vi "UiGasMeasurement.vi"() -> ()   [LabVIEW 2011]
uses:
  Output - Cluster b2g1.ctl
  <vilib>/Platform/TimedLoop/XDataNode/timing_clust.ctl
  <vilib>/Platform/TimedLoop/XDataNode/nitl_modes.ctl
  <vilib>/Platform/TimedLoop/XDataNode/wakeup.ctl
  <vilib>/Instr/_visa.llb/VISA Configure Serial Port (Instr).vi
  <vilib>/Platform/TimedLoop/XDataNode/XDataNode.xnode
  <vilib>/Platform/TimedLoop/XDataNode/XDNodeRunTimeDep.lvlib
panel:
  out "Verlauf":T1(graph)
  out "pump":bool
  out "timestamp 2":timestamp
  out "log":string[](array[string])
  out "h2":dbl
  out "ch4":dbl
  out "co2":dbl
  out "timestamp":timestamp
  out "return count":u32
  out "read string":string
  out "Volumen [l]":dbl format="%.2f"
  in  "stop":bool
  out "TS-6 [°C]":dbl format="%.2g"
  out "DS-3 [bar]":dbl format="%.5g"
  # "#MS 26.07.12 15:36:48    21.98 Vol% CO2  72.54 Vol% CH4   1.05 Vol% H2\n\n#AL 27.07.12 16:34:22  37 EIN externe Pumpe \n\n#AL 27.07.12 16:40:29  37 AUS externe Pumpe"
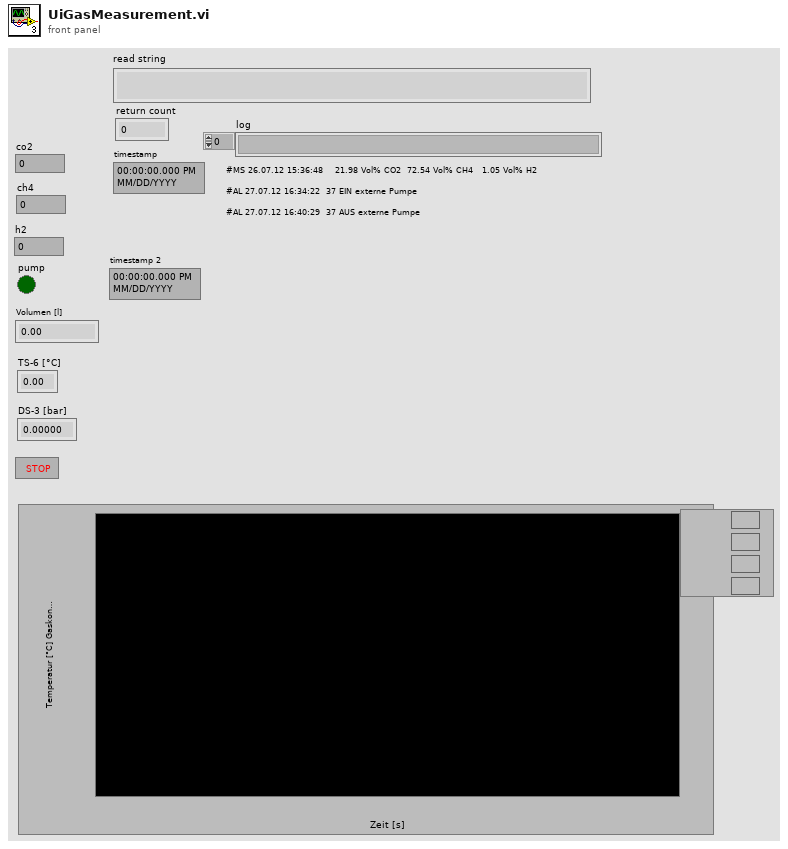
[diagram p1: front panel]
types:
  T1 = cluster{"co2 [%]":dbl, "ch4 [%]":dbl, "h2 [%]":dbl, "TS-6 [°C]":dbl}
  T2 = cluster{"ch4 [%]":dbl, "co2 [%]":dbl, "h2 [%]":dbl, "pump":bool, "log":string[], "Volumen [l]":dbl, "TS-6 [°C]":dbl, "DS-3 [bar]":dbl}
  T3 = typedef "Output - Cluster b2g1.ctl" = cluster{"DFS-1 [dl]":u64, "FS-3 [l]":dbl, "DFS-1 [l/min]":dbl, "DS-1 [bar]":dbl, "V-10 ZU":bool, "V-14 ZU":bool, "FS-1 [l]":dbl, "FS-2 [l]":dbl, "TS-4 [°C]":dbl, "HS-1":bool, "V-13 [%]":u8, "V-15 [%]":u8, "P-4 [%]":u8, "P-5 [%]":u8, "Dosierung":bool, "MR Max Füllstand":bool, "MR Min Füllstand":bool, "Dosiermenge [l]":sgl, "V-14 AUF":bool, "V-10 AUF":bool, "T-1 Max Füllstand":bool, "T-1 Min Füllstand":bool, "T-2 Max Füllstand":bool, "T-2 Min Füllstand":bool, "pHS-1 [pH]":dbl, "P-4 RUN":bool, "P-5 RUN ":bool, "V-33 AUF":bool, "V-33 ZU":bool, "V-34 AUF":bool, "V-34 ZU":bool, "P-4 ERR":bool, "P-5 ERR":bool, "TS-5 [°C]":dbl, "GZ-1 [dl]":u64, "TS-6 [°C]":dbl, "DS-3 [bar]":dbl}
  T4 = typedef "XDNodeRunTimeDep.lvlib/timing_clust.ctl" = cluster{"Expected End [f-1]":u64, "Actual End [f-1]":u64, "Finished Late? [f-1]":bool, "Expected End [i-1]":u64, "Actual End [i-1]":u64, "Finished Late? [i-1]":bool, "Expected Start [i]":u64, "Actual Start [i]":u64, "Expected Start [f]":u64, "Actual Start [f]":u64, "Source Name":string, "Structure Name":string, "Period":i64, "Deadline":i64, "Offset":i64, "Start":i64, "Priority":i32, "Timeout":i32, "Mode":T5, "Wakeup Reason":T6, "Error":errorcluster, "Source Type":string, "Secondary Source Type":string, "Global End Time":u64, "Global Start Time":u64, "Frame Duration":u64, "Iteration Duration":u64, "Assigned CPU":i32, "I/O Scan Engine Mode":u32}
  T5 = typedef "XDNodeRunTimeDep.lvlib/nitl_modes.ctl" = enum32{"No Change", "Process missed periods, maintain original phase", "Discard missed periods, maintain original phase", "Process missed periods, ignore original phase", "Discard missed periods, ignore original phase"}
  T6 = typedef "XDNodeRunTimeDep.lvlib/wakeup.ctl" = enum32{"Normal", "Aborted", "Asynchronous wakeup", "Timing source error", "Timed loop error", "Timeout"}
  T7 = enum32{"invalid app kind", "Development System", "Run Time System", "Student Edition", "Embedded LabVIEW", "Evaluation", "Custom"}
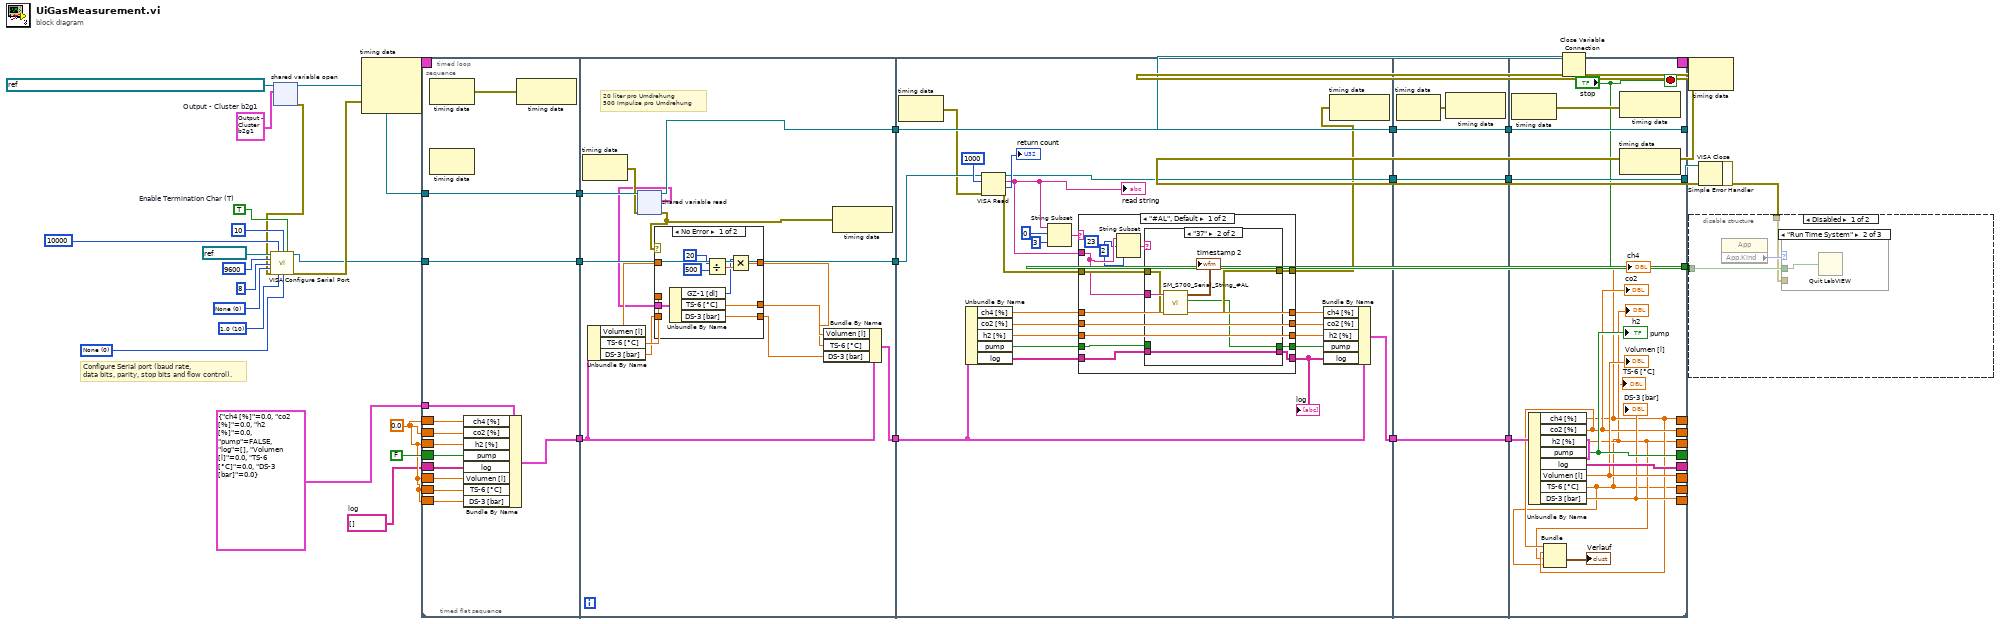
[diagram p0: block diagram]
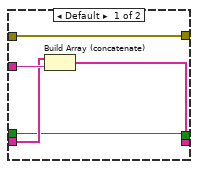
[diagram p6: hidden frame]
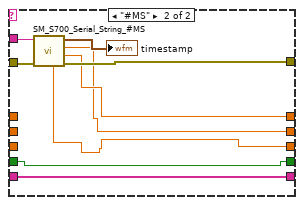
[diagram p7: hidden frame]
diagram:
  w1 = string[] []  # log
  w2 = 0.0 ("co2")
  w17 = u16 0 items=["None", "Odd", "Even", "Mark", "Space"] ("parity")
  w14 = u16 10 items=["1.0"=10, "1.5"=15, "2.0"=20] ("stop bits")
  w13 = u16 0 items=["None"=0, "XON/XOFF"=1, "RTS/CTS"=2, "DTR/DSR"=4] ("flow control")
  w15 = TRUE  # Enable Termination Char (T)
  w26 = T3 {"DFS-1 [dl]"=0, "FS-3 [l]"=0.0, "DFS-1 [l/min]"=0.0, "DS-1 [bar]"=0.0, "V-10 ZU"=FALSE, "V-14 ZU"=FALSE, "FS-1 [l]"=0.0, "FS-2 [l]"=0.0, "TS-4 [°C]"=0.0, "HS-1"=FALSE, "V-13 [%]"=0, "V-15 [%]"=0, "P-4 [%]"=0, "P-5 [%]"=0, "Dosierung"=FALSE, "MR Max Füllstand"=FALSE, "MR Min Füllstand"=FALSE, "Dosiermenge [l]"=0.0, "V-14 AUF"=FALSE, "V-10 AUF"=FALSE, "T-1 Max Füllstand"=FALSE, "T-1 Min Füllstand"=FALSE, "T-2 Max Füllstand"=FALSE, "T-2 Min Füllstand"=FALSE, "pHS-1 [pH]"=0.0, "P-4 RUN"=FALSE, "P-5 RUN "=FALSE, "V-33 AUF"=FALSE, "V-33 ZU"=FALSE, "V-34 AUF"=FALSE, "V-34 ZU"=FALSE, "P-4 ERR"=FALSE, "P-5 ERR"=FALSE, "TS-5 [°C]"=0.0, "GZ-1 [dl]"=0, "TS-6 [°C]"=0.0, "DS-3 [bar]"=0.0}  # Output - Cluster b2g1
  # "Configure Serial port (baud rate,\ndata bits, parity, stop bits and flow control)."
  n1 = shared-variable-open(refnum<k21> "ni.var.psp://10.27.40.24/variables - b2g1/data - network - b2g1" ("shared variable refnum in"), w26) -> (w27:refnum<k21>, w10:errorcluster)  [unwired: 2 in]
  n2 = call-poly "VISA Configure Serial Port"("VISA resource name"=refnum<visa-resource-name> "COM1", "timeout (10sec)"=u32 10000, "termination char\n(0xA = '\\n' = LF)"=u8 10 ("termination char\n(0xA = '\\n' = LF)"), "Enable Termination\nChar (T)"=w15, "baud rate (9600)"=u32 9600 ("baud rate"), "data bits (8)"=u16 8 ("data bits"), "parity (0:none)"=w17, "error in (no error)"=w10, "stop bits (10: 1 bit)"=w14, "flow control (0:none)"=w13) -> ("VISA resource name out"=w6:refnum<visa-resource-name>, "error out"=w9:errorcluster)  [unwired: 4 in]
  n3 = node-c288(w9) -> (w25:T4)  [unwired: 2 in]
  n4 = timed-loop {
    timing: w25 -> [_]
    timing-out: [_] -> w24
    tunnel: w27 -> [w50]
    tunnel: [w49] -> w22
    tunnel: [w48] -> w21
    tunnel: w6 -> [w47]
    tunnel: [w46] -> w5
    shift-right: [w45] -> _
    shift-left: w1 -> [w44]
    tunnel: T2 {"ch4 [%]"=0.0, "co2 [%]"=0.0, "h2 [%]"=0.0, "pump"=FALSE, "log"=[], "Volumen [l]"=0.0, "TS-6 [°C]"=0.0, "DS-3 [bar]"=0.0} ("Cluster") -> [w43]
    shift-right: [w42] -> _
    shift-left: w2 -> [w41]
    shift-right: [w40] -> _
    shift-left: w2 -> [w39]
    shift-right: [w38] -> _
    shift-left: w2 -> [w37]
    shift-right: [w36] -> _
    shift-left: FALSE ("pump") -> [w35]
    shift-right: [w34] -> _
    shift-left: w2 -> [w33]
    shift-right: [w32] -> _
    shift-left: w2 -> [w31]
    shift-right: [w30] -> _
    shift-left: w2 -> [w29]
    stop <- "stop" stop-if-true
    n5 = timed-sequence {
      timing: _ -> [_]
      timing-out: _ -> [_]
      tunnel: w50 -> [w84]
      tunnel: [w83] -> w49
      tunnel: [w82] -> w48
      tunnel: w47 -> [w79]
      tunnel: [w78] -> w46
      tunnel: [w77] -> w45
      tunnel: w44 -> [w76]
      tunnel: w43 -> [w73]
      tunnel: [w70] -> w42
      tunnel: w41 -> [w69]
      tunnel: [w68] -> w40
      tunnel: w39 -> [w67]
      tunnel: [w66] -> w38
      tunnel: w37 -> [w65]
      tunnel: [w64] -> w36
      tunnel: w35 -> [w63]
      tunnel: [w62] -> w34
      tunnel: w33 -> [w61]
      tunnel: [w60] -> w32
      tunnel: w31 -> [w59]
      tunnel: [w58] -> w30
      tunnel: w29 -> [w57]
      n6 = timed-flat-sequence {
        tunnel: w76 -> [w88]
        tunnel: w79 -> [w96]
        tunnel: w84 -> [w97]
        tunnel: [w97] -> w75
        tunnel: [w96] -> w74
        tunnel: w73 -> [w94]
        tunnel: [w93] -> w71
        tunnel: w69 -> [w92]
        tunnel: w67 -> [w91]
        tunnel: w65 -> [w90]
        tunnel: w63 -> [w89]
        tunnel: w61 -> [w85]
        tunnel: w59 -> [w86]
        tunnel: w57 -> [w87]
        tunnel: [w114] -> w81
        tunnel: [w113] -> w80
        tunnel: w75 -> [w116]
        tunnel: w74 -> [w113]
        tunnel: [w111] -> w72
        tunnel: w71 -> [w110]
        tunnel: w81 -> [w156]
        tunnel: w80 -> [w153]
        tunnel: w72 -> [w143]
        tunnel: [w156] -> w56
        tunnel: [w152] -> w54
        tunnel: [w142] -> w52
        tunnel: w56 -> [w198]
        tunnel: [w198] -> w55
        tunnel: w54 -> [w197]
        tunnel: [w197] -> w53
        tunnel: w52 -> [w196]
        tunnel: [w196] -> w51
        tunnel: [w211] -> w64
        tunnel: [w205] -> w66
        tunnel: [w207] -> w68
        tunnel: [w206] -> w70
        tunnel: [w212] -> w77
        tunnel: [w216] -> w78
        tunnel: ["stop"] -> w82
        tunnel: [w217] -> w83
        tunnel: w55 -> [w217]
        tunnel: w53 -> [w216]
        tunnel: w51 -> [w213]
        tunnel: [w209] -> w62
        tunnel: [w204] -> w60
        tunnel: [w210] -> w58
        frame #0 {
          n7 = node-c288() -> (w95:errorcluster)  [unwired: 1 in]
          n8 = Bundle By Name(cluster=w94, "ch4 [%]"=w92, "co2 [%]"=w91, "h2 [%]"=w90, "pump"=w89, "log"=w88, "Volumen [l]"=w87, "TS-6 [°C]"=w86, "DS-3 [bar]"=w85) -> (w93:T2)
          n9 = node-c288(w95) -> ()  [unwired: 1 out]
        }
        frame #1 {
          # "20 liter pro Umdrehung\n500 Impulse pro Umdrehung"
          n10 = node-c288() -> (w115:errorcluster)  [unwired: 1 in]
          n11 = Unbundle By Name(w110) -> ("Volumen [l]"=w108:dbl, "TS-6 [°C]"=w106:dbl, "DS-3 [bar]"=w104:dbl)
          n12 = shared-variable-read(w116, w115) -> (w114:refnum<k21>, w112:errorcluster, w103:T3)  [unwired: 1 out]
          n13 = case shown="No Error" w112 {
            tunnel: [w117 w127] -> w109
            tunnel: w108 -> [_ w127]
            tunnel: [w118 w126] -> w107
            tunnel: w106 -> [_ w126]
            tunnel: [w119 w125] -> w105
            tunnel: w104 -> [_ w125]
            tunnel: w103 -> [w120 _]
            frame No Error {
              n14 = Unbundle By Name(w120) -> ("GZ-1 [dl]"=w121:u64, "TS-6 [°C]"=w118:dbl, "DS-3 [bar]"=w119:dbl)
              n15 = Divide(x=20, y=500) -> (x/y=w124:dbl)
              n16 = Multiply(x=w121, y=w124) -> (x*y=w117:dbl)
            }
            frame Error {
            }
          }
          n17 = Bundle By Name(cluster=w110, "Volumen [l]"=w109, "TS-6 [°C]"=w107, "DS-3 [bar]"=w105) -> (w111:T2)
          n18 = node-c288(w112) -> ()  [unwired: 1 out]
        }
        frame #2 {
          n19 = node-c288() -> (w151:errorcluster)  [unwired: 1 in]
          n20 = Unbundle By Name(w143) -> ("ch4 [%]"=w140:dbl, "co2 [%]"=w139:dbl, "h2 [%]"=w138:dbl, "pump"=w137:bool, "log"=w144:string[])
          n21 = VISA Read(VISA resource name=w153, byte count=u32 1000 ("bytes to read"), error in (no error)=w151) -> (VISA resource name out=w152:refnum<visa-resource-name>, read buffer=w147:string, return count=→"return count":u32, error out=w150:errorcluster)
          "read string" <- w147
          n22 = String Subset(string=w147, offset (0)=0, length (rest)=3 ("length (rest)")) -> (substring=w146:string)
          n23 = case shown="\"#AL\", Default" w146 {
            tunnel: w150 -> [w167 w189]
            tunnel: [w166 w188] -> w149
            tunnel: w147 -> [w165 w187]
            tunnel: [w168 w186] -> w141
            tunnel: w144 -> [w169 w186]
            tunnel: w140 -> [w163 _]
            tunnel: w139 -> [w162 _]
            tunnel: w138 -> [w161 _]
            tunnel: w137 -> [w160 w181]
            tunnel: [w163 w184] -> w136
            tunnel: [w162 w183] -> w135
            tunnel: [w161 w182] -> w134
            tunnel: [w159 w181] -> w133
            frame "#AL", Default {
              n24 = String Subset(string=w165, offset (0)=23, length (rest)=2 ("length (rest)")) -> (substring=w158:string)
              n25 = case shown="\"37\"" w158 {
                tunnel: w165 -> [w174 w179]
                tunnel: w169 -> [w173 w180]
                tunnel: [w172 w180] -> w168
                tunnel: w167 -> [w171 w178]
                tunnel: [w171 w177] -> w166
                tunnel: w160 -> [w170 _]
                tunnel: [w170 w175] -> w159
                frame Default {
                  n26 = Build Array (concatenate)(w173, w174) -> (w172:string[])
                }
                frame "37" {
                  n27 = call "SM_S700_Serial_String_#AL.vi"("error in (no error)"=w178, "read buffer"=w179) -> ("error out"=w177:errorcluster, "pump"=w175:bool, "timestamp"=→"timestamp 2":timestamp)  [unwired: 7 in]
                }
              }
            }
            frame "#MS" {
              n28 = call "SM_S700_Serial_String_#MS.vi"("error in (no error)"=w189, "read buffer"=w187) -> ("error out"=w188:errorcluster, "ch4"=w184:dbl, "co2"=w183:dbl, "timestamp"=→"timestamp":timestamp, "h2"=w182:dbl)  [unwired: 5 in]
            }
          }
          "log" <- w141
          n29 = Bundle By Name(cluster=w143, "ch4 [%]"=w136, "co2 [%]"=w135, "h2 [%]"=w134, "pump"=w133, "log"=w141) -> (w142:T2)
          n30 = node-c288(w149) -> ()  [unwired: 1 out]
        }
        frame #3 {
          n31 = node-c288() -> (w195:errorcluster)  [unwired: 1 in]
          n32 = node-c288(w195) -> ()  [unwired: 1 out]
        }
        frame #4 {
          n33 = node-c288() -> (w215:errorcluster)  [unwired: 1 in]
          n34 = Unbundle By Name(w213) -> ("ch4 [%]"=w206:dbl, "co2 [%]"=w207:dbl, "h2 [%]"=w205:dbl, "pump"=w211:bool, "log"=w212:string[], "Volumen [l]"=w210:dbl, "TS-6 [°C]"=w204:dbl, "DS-3 [bar]"=w209:dbl)
          "pump" <- w211
          "DS-3 [bar]" <- w209
          "TS-6 [°C]" <- w204
          "Volumen [l]" <- w210
          "co2" <- w207
          "ch4" <- w206
          "h2" <- w205
          n35 = Bundle("co2 [%]"=w207, "ch4 [%]"=w206, "h2 [%]"=w205, "TS-6 [°C]"=w204) -> (→"Verlauf":T1)  [unwired: 1 in]
          n36 = node-c288(w215) -> ()  [unwired: 1 out]
        }
      }
    }
    n37 = node-c288() -> ()  [unwired: 1 in, 1 out]
    n38 = node-c288() -> ()  [unwired: 1 in, 1 out]
  }
  n39 = node-c288(w24) -> (w23:errorcluster)
  n40 = Close Variable Connection(8:w23, 11:w22) -> (0:w8:errorcluster)
  n41 = VISA Close(VISA resource name=w5, error in (no error)=w8) -> (error out=w18:errorcluster)
  n42 = call <vilib>:"Simple Error Handler.vi"("error in (no error)"=w18) -> ("error out"=w7:errorcluster)  [unwired: 4 in, 4 out]
  n43 = disable-structure shown="Disabled" {
    disable-tunnel: w21 -> [w226 _]
    disable-tunnel: w7 -> [w225 _]
    frame Disabled {
      n44 = property class="App"() -> ("App.Kind"=w227:T7)  [unwired: 2 in, 2 out]
      n45 = case shown="\"Run Time System\"" w227 {
        tunnel: w226 -> [_ w228 _]
        tunnel: w225 -> [_ _ _]
        frame "invalid app kind", Default {
        }
        frame "Run Time System" {
          n46 = Quit LabVIEW(quit? (T)=w228) -> ()
        }
        frame "Development System" {
        }
      }
    }
    frame Enabled {
    }
  }
